vi "playlist.vi"() -> ()   [LabVIEW 2020]
panel:
  out "Array":string[][](array[string])=[["Sensor 1", "Sensor 2", "Sensor 3", "Song"], ["0", "0", "0", "Pyar"], ["0", "0", "1", "Chali"], ["0", "1", "0", "Dil"], ["0", "1", "1", "Aplam"], ["1", "0", "0", "Love"], ["1", "0", "1", "Inkem "], ["1", "1", "0", "Gira"]]
  in  "Sensor 3":bool
  in  "Sensor 2":bool
  in  "Sensor 1":bool
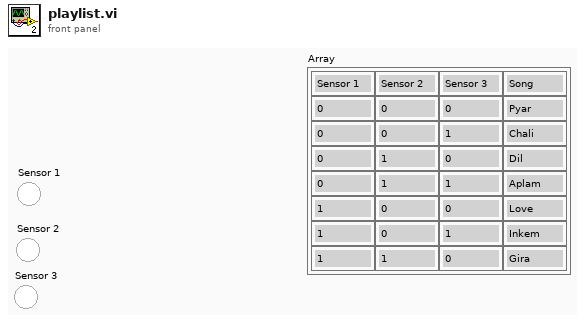
[diagram p1: front panel]
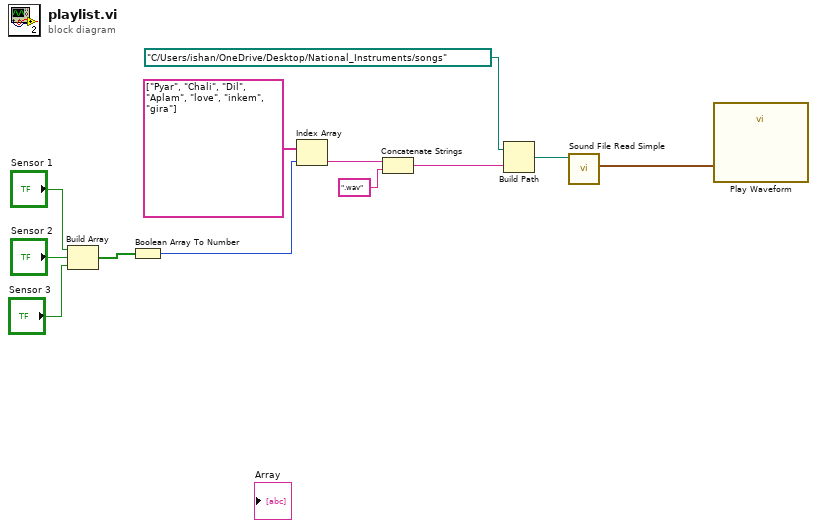
[diagram p0: block diagram]
diagram:
  n1 = Build Array "Build Array"("Sensor 1", "Sensor 2", "Sensor 3") -> (w5:bool[])
  n2 = Boolean Array To Number(Boolean array=w5) -> (number=w2:u32)
  n3 = Index Array "Index Array"(array=string[] ["Pyar", "Chali", "Dil", "Aplam", "love", "inkem", "gira"], index=w2) -> (element=w4:string)
  n4 = Concatenate Strings "Concatenate Strings"(w4, ".wav") -> (w9:string)
  n5 = Build Path(base path=path "C:/Users/ishan/OneDrive/Desktop/National_Instruments/songs" ("path"), name or relative path=w9) -> (appended path=w8:path)
  n6 = call <vilib>:"Sound File Read Simple.vi"("path"=w8) -> ("data"=w12:waveform(dbl)[])  [unwired: 7 in, 3 out]
  n7 = call "Play Waveform"("Data"=w12) -> ()  [unwired: 18 in, 1 out]
